vi "Perform Action.vi"(8 "Error In":errorcluster, 10 "Input":variant, 11 "reference in":refnum<class "Instr Base.lvclass">) -> (0 "Error Out":errorcluster, 2 "Output":variant, 3 "reference out":refnum<class "Instr Base.lvclass">)   [LabVIEW 2023, in "HAL GOOP4.lvlib" / "Instr Base.lvclass"]
uses:
  Instr Base.lvclass
  Interfaces/IConfigure/IConfigure.lvclass
  Instr Base.lvclass/Instr Base.ctl
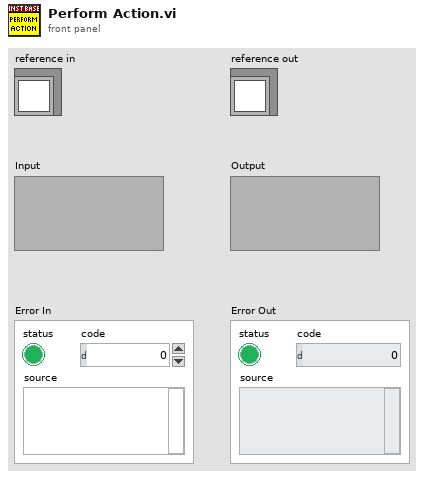
[diagram p1: front panel]
types:
  T1 = typedef "HAL GOOP4.lvlib/Instr Base.lvclass/ObjectAttributes.ctl" = cluster{"IConfigure":refnum<class "IConfigure.lvclass">, "Ref Count":u8}
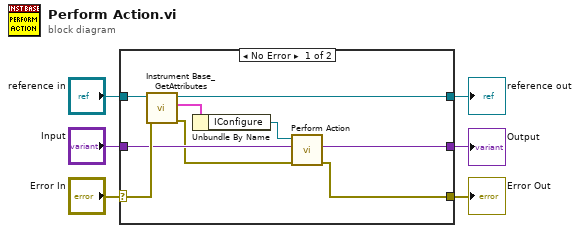
[diagram p0: block diagram]
diagram:
  n1 = case shown="No Error" "Error In" {
    selector: "Error In" -> [w15 w17]
    tunnel: [w8 w17] -> w5
    tunnel: [w12 w16] -> w3
    tunnel: "reference in" -> [w13 w16]
    tunnel: "Input" -> [w10 _]
    tunnel: [w7 _] -> w1
    frame No Error {
      n2 = call "Instrument Base_GetAttributes.vi"("Error In"=w15, "reference in"=w13) -> ("Error Out"=w9:errorcluster, "Data"=w14:T1, "reference out"=w12:refnum<class "Instr Base.lvclass">)  [unwired: 6 in, 1 out]
      n3 = Unbundle By Name(w14) -> ("IConfigure"=w11:refnum<class "IConfigure.lvclass">)
      n4 = call-dynamic "Perform Action.vi"("error in (no error)"=w9, "Input"=w10, "IConfigure in"=w11) -> ("error out"=w8:errorcluster, "Output"=w7:variant)  [unwired: 6 in, 1 out]
    }
    frame Error {
    }
  }
  "Error Out" <- w5
  "reference out" <- w3
  "Output" <- w1
